vi "CVT2NamedReadTest.vi"() -> (3 "Unit Test Framework Results":T1)   [LabVIEW 2014, in "UnitTests.lvlib"]
uses:
  UnitTests.lvlib
  <vilib>/utf/common/utf_test_result_troll.ctl
  <vilib>/utf/common/utf_test_result.ctl
  <vilib>/utf/common/utf_test_result_failure.ctl
  <vilib>/utf/common/utf_test_comparison_operators.ctl
  <vilib>/utf/common/utf_vi_tag.ctl
  dev/source/vi.lib/NI/Current Value Table/DataTypes/I32_Read.vi
  dev/source/vi.lib/NI/Current Value Table/Type to Enum.vi
  dev/source/vi.lib/NI/Current Value Table/DataTypes/I32_Type To Enum.vi
  dev/source/vi.lib/NI/Current Value Table/Memory Block.vi
  dev/source/vi.lib/NI/Current Value Table/DataTypes/I32_Memory Block.vi
  dev/source/vi.lib/NI/Current Value Table/FGVs/Tag Memory.vi
  dev/source/vi.lib/NI/Current Value Table/FGVs/CVT Globals.vi
  <vilib>/utf/NI_UnitTestFramework.lvlib
  dev/source/vi.lib/NI/Current Value Table/Current Value Table.lvlib
panel:
  out "Value":i32
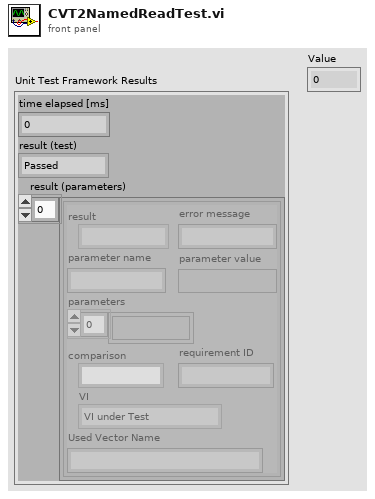
[diagram p1: front panel]
types:
  T1 = typedef "NI_UnitTestFramework.lvlib/utf_test_result_troll.ctl" = cluster{"time elapsed [ms]":u32, "result (test)":T2, "result (parameters)":T3[]}
  T2 = typedef "NI_UnitTestFramework.lvlib/utf_test_result.ctl" = enum16{"Passed", "Failed", "Error", "Skipped", "Not Processed"}
  T3 = typedef "NI_UnitTestFramework.lvlib/utf_test_result_failure.ctl" = cluster{"result":T2, "error message":string, "parameter name":string, "parameter value":variant, "parameters":variant[], "comparison":T4, "requirement ID":string, "VI":T5, "Used Vector Name":string}
  T4 = typedef "NI_UnitTestFramework.lvlib/utf_test_comparison_operators.ctl" = enum16{"=", "!=", ">", ">=", "<", "<=", "range", "symmetric tolerance", "asymmetric tolerance", "string contains", "string not contain", "array size", "string length", "array range", "by element", "array range (limit array)", "user-defined", "array contains", "array not contain", "vector length", "= (elm)", "!= (elm)", "= (case insensitive)", "!= (case insensitive)"}
  T5 = typedef "NI_UnitTestFramework.lvlib/utf_vi_tag.ctl" = enum16{"Setup VI", "VI under Test", "Teardown VI"}
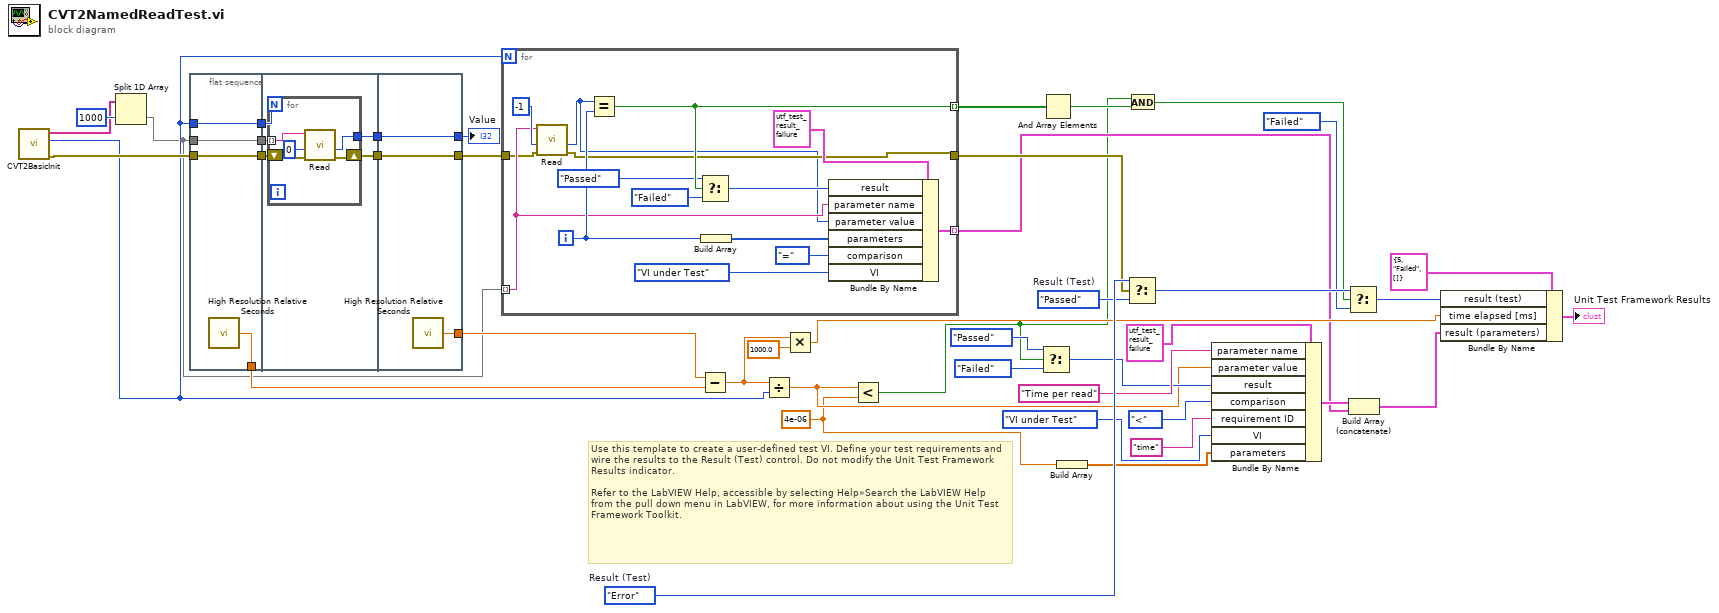
[diagram p0: block diagram]
diagram:
  w13 = 4e-06 ("y")
  w38 = utf_test_result."Error"  # Result (Test)
  w37 = utf_test_result."Passed"  # Result (Test)
  # "Use this template to create a user-defined test VI. Define your test requirements and wire the results to the Result (Test) control. Do not modify the Unit Test Framework Results indicator. \n\nRefer to the LabVIEW Help, accessible by selecting Help»Search the LabVIEW Help from the pull down menu in LabVIEW, for more information about using the Unit Test Framework Toolkit."
  n1 = call "CVT2BasicInit.vi"() -> ("error out"=w6:errorcluster, "Tags per type out"=w5:i32, "names"=w2:string[])  [unwired: 9 in]
  n2 = Split 1D Array(array=w2, index=1000) -> (second subarray=w1:string[])  [unwired: 1 out]
  n3 = flat-sequence {
    tunnel: [w47] -> w40
    tunnel: w6 -> [w45]
    tunnel: [w46] -> w32
    tunnel: w5 -> [w46]
    tunnel: [w45] -> w31
    tunnel: [w44] -> w4
    tunnel: w1 -> [w44]
    tunnel: w32 -> [w52]
    tunnel: w31 -> [w51]
    tunnel: [w50] -> w30
    tunnel: [w49] -> w8
    tunnel: w4 -> [w48]
    tunnel: [w60] -> w41
    tunnel: w30 -> [w59]
    tunnel: [w59] -> w27
    tunnel: [w58] -> w7
    tunnel: w8 -> [w58]
    frame #0 {
      n4 = call <vilib>:"High Resolution Relative Seconds.vi"() -> ("relative seconds"=w47:dbl)
    }
    frame #1 {
      n5 = for {
        N: w52 -> [_]
        shift-right: [w56] -> w50
        shift-left: w51 -> [w57]
        tunnel: [w55] -> w49
        tunnel: w48 -> [w53] mode=indexing
        n6 = call-poly "Read.vi"("error in (no error)"=w57, "Default"=0, "Tag Name"=w53) -> ("error out"=w56:errorcluster, "Value"=w55:i32)  [unwired: 7 in]
      }
    }
    frame #2 {
      n7 = call <vilib>:"High Resolution Relative Seconds.vi"() -> ("relative seconds"=w60:dbl)
    }
  }
  n8 = for {
    N: w5 -> [_]
    tunnel: w1 -> [w64] mode=indexing
    tunnel: w27 -> [w63]
    tunnel: [w62] -> w26
    tunnel: [w73] -> w25 mode=indexing
    tunnel: [w69] -> w11 mode=indexing
    i -> [w66]
    n9 = call-poly "Read.vi"("error in (no error)"=w63, "Default"=-1, "Tag Name"=w64) -> ("error out"=w62:errorcluster, "Value"=w61:i32)  [unwired: 7 in]
    n10 = Equal?(x=w61, y=w66) -> (x = y?=w73:bool)
    n11 = Select(t=utf_test_result."Passed" ("result"), s=w73, f=utf_test_result."Failed" ("result")) -> (s? t:f=w70:T2)
    n12 = Build Array(w66) -> (w67:i32[])
    n13 = Bundle By Name(cluster=T3 {"result"=enum."Passed", "error message"="", "parameter name"="", "parameter value"=variant, "parameters"=[], "comparison"=enum."=", "requirement ID"="", "VI"=enum."Setup VI", "Used Vector Name"=""} ("Unit Test Framework - result (parameters)"), "result"=w70, "parameter name"=w64, "parameter value"=w61, "parameters"=w67, "comparison"=utf_test_comparison_operators."=", "VI"=utf_vi_tag."VI under Test") -> (w69:T3)
  }
  n14 = Subtract(x=w41, y=w40) -> (x-y=w29:dbl)
  n15 = Divide(x=w29, y=w5) -> (x/y=w16:dbl)
  n16 = Multiply(x=w29, y=1000.0) -> (x*y=w33:dbl)
  n17 = Less?(x=w16, y=w13) -> (x < y?=w9:bool)
  n18 = Select(t=utf_test_result."Passed" ("result"), s=w9, f=utf_test_result."Failed" ("result")) -> (s? t:f=w17:T2)
  n19 = And Array Elements(Boolean array=w25) -> (logical AND=w24:bool)
  n20 = Build Array(w13) -> (w12:dbl[])
  n21 = Select(t=w38, s=w26, f=w37) -> (s? t:f=w23:T2)
  n22 = And(x=w9, y=w24) -> (x .and. y?=w10:bool)
  n23 = Bundle By Name(cluster=T3 {"result"=enum."Passed", "error message"="", "parameter name"="", "parameter value"=variant, "parameters"=[], "comparison"=enum."=", "requirement ID"="", "VI"=enum."Setup VI", "Used Vector Name"=""} ("Unit Test Framework - result (parameters)"), "parameter name"="Time per read", "parameter value"=w16, "result"=w17, "comparison"=utf_test_comparison_operators."<", "requirement ID"="time", "VI"=utf_vi_tag."VI under Test", "parameters"=w12) -> (w36:T3)
  n24 = Select(t=w23, s=w10, f=utf_test_result."Failed") -> (s? t:f=w21:T2)
  n25 = Build Array (concatenate)(w36, w11) -> (w35:T3[])
  n26 = Bundle By Name(cluster=T1 {"time elapsed [ms]"=5, "result (test)"=enum."Failed", "result (parameters)"=[]} ("Unit Test Framework - Result"), "result (test)"=w21, "time elapsed [ms]"=w33, "result (parameters)"=w35) -> (→"Unit Test Framework Results":T1)
  "Value" <- w7
